vi "Build Status Message.vi"(5 "Macro Repeat":i32, 7 "Step Repeat":i32, 8 "error in (no error)":errorcluster, 9 "Start Time":timestamp, 10 "Step":i32, 11 "Macro in":refnum<class "Macro.lvclass">) -> (0 "error out":errorcluster, 2 "Status":string, 3 "Macro out":refnum<class "Macro.lvclass">)   [LabVIEW 2020, in "MacroAssert.lvlib" / "Macro.lvclass"]
uses:
  Macro.lvclass
  Step/Step.lvclass
  Macro.lvclass/Macro.ctl
  <userlib>/_OpenG.lib/array/array.llb/openg_array.lvlib
  <userlib>/_OpenG.lib/array/array.llb/Filter 1D Array with Scalar (String)__ogtk.vi
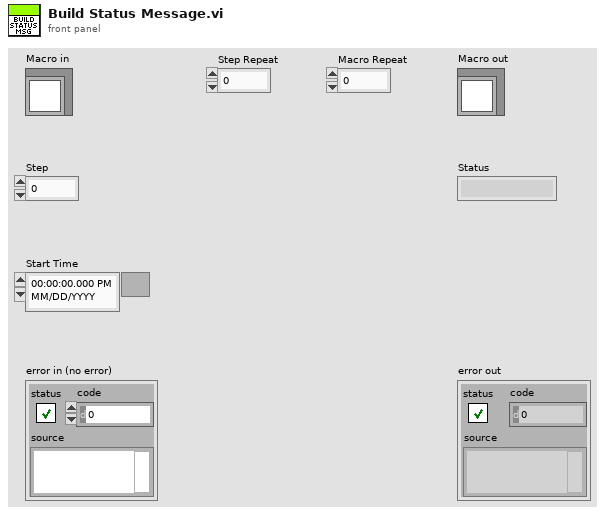
[diagram p1: front panel]
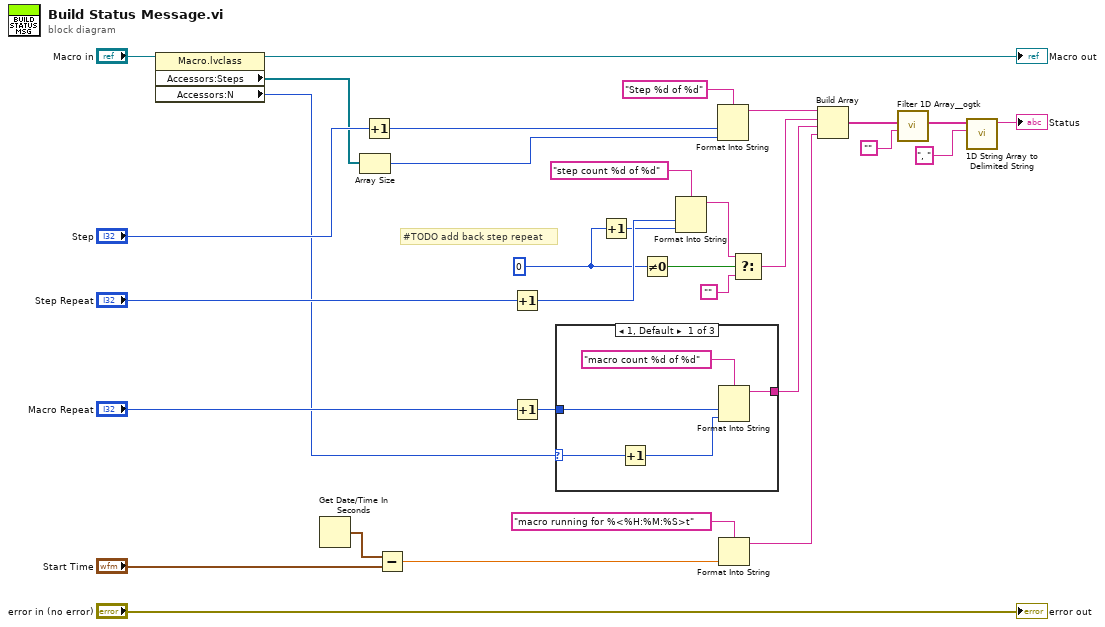
[diagram p0: block diagram]
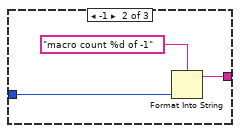
[diagram p2: hidden frame]
diagram:
  w1 = 0 ("Repeat")
  # "#TODO add back step repeat"
  n1 = property class="Macro.lvclass"(reference="Macro in") -> (reference out=→"Macro out":refnum<class "Macro.lvclass">, "Accessors:Steps"=w2:refnum<class "Step.lvclass">[], "Accessors:N"=w3:i32)  [unwired: 1 in, 1 out]
  n2 = Get Date/Time In Seconds() -> (seconds since 1Jan1904=w17:timestamp)
  n3 = Array Size(array=w2) -> (size(s)=w26:i32)
  n4 = Increment(x="Step") -> (x+1=w24:i32)
  n5 = Subtract(x=w17, y="Start Time") -> (x-y=w15:dbl)
  n6 = Increment(x="Step Repeat") -> (x+1=w23:i32)
  n7 = Increment(x="Macro Repeat") -> (x+1=w19:i32)
  n8 = case shown="1, Default" w3 {
    selector: w3 -> [w34 _ _]
    tunnel: w19 -> [w36 w39 _]
    tunnel: [w35 w38 _] -> w12
    frame 1, Default {
      n9 = Increment(x=w34) -> (x+1=w33:i32)
      n10 = Format Into String(format string="macro count %d of %d", w36, w33) -> (resulting string=w35:string)  [unwired: 2 in, 1 out]
    }
    frame -1 {
      n11 = Format Into String(format string="macro count %d of -1", w39) -> (resulting string=w38:string)  [unwired: 2 in, 1 out]
    }
    frame 0 {
    }
  }
  n12 = Increment(x=w1) -> (x+1=w22:i32)
  n13 = Not Equal To 0?(x=w1) -> (x != 0?=w28:bool)
  n14 = Format Into String(format string="step count %d of %d", w23, w22) -> (resulting string=w21:string)  [unwired: 2 in, 1 out]
  n15 = Format Into String(format string="Step %d of %d", w24, w26) -> (resulting string=w14:string)  [unwired: 2 in, 1 out]
  n16 = Format Into String(format string="macro running for %<%H:%M:%S>t", w15) -> (resulting string=w11:string)  [unwired: 2 in, 1 out]
  n17 = Select(t=w21, s=w28, f="") -> (s? t:f=w13:string)
  n18 = Build Array(w14, w13, w12, w11) -> (w10:string[])
  n19 = call-poly <userlib>:"Filter 1D Array__ogtk.vi"("items to filter"="", "array"=w10) -> ("filtered array"=w8:string[])  [unwired: 4 in, 1 out]
  n20 = call <vilib>:"1D String Array to Delimited String.vi"("delimiter"=", " ("Separator (,)"), "string array"=w8) -> ("delimited string"=→"Status":string)  [unwired: 9 in]
  "error out" <- "error in (no error)"
